vi "Smart_Irrigation_Labview.vi"() -> ()   [LabVIEW 2020]
panel:
  in  "Table Control":string[][](table)
  out "Moisture Sensor":dbl(graph)
  out "Flow Out":bool
  out "Moisture-Level":dbl(knob) scale=0.0..100.0
  out "Water-level Sensor":dbl(graph)
  in  "VISA Resource Port":refnum<visa-resource-name>
  out "PUMP ON":bool
  out "PUMP  OFF":bool
  out "Tank (Liters/sec)":dbl(slide) scale=0.0..100.0
  # "RAGING BULLS"
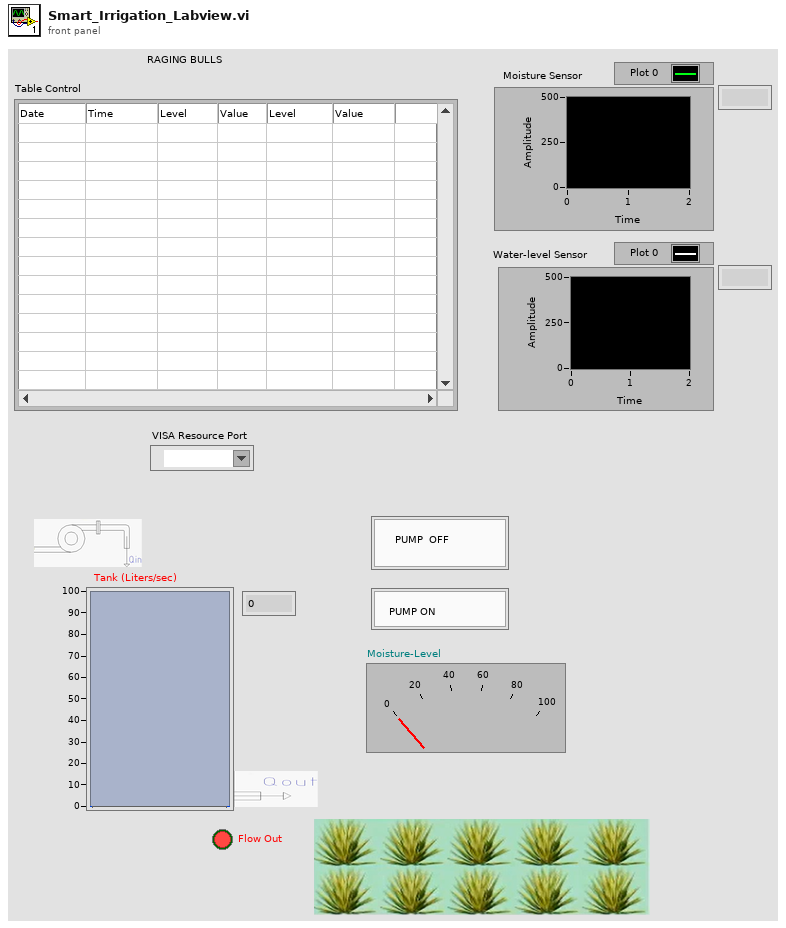
[diagram p1: front panel]
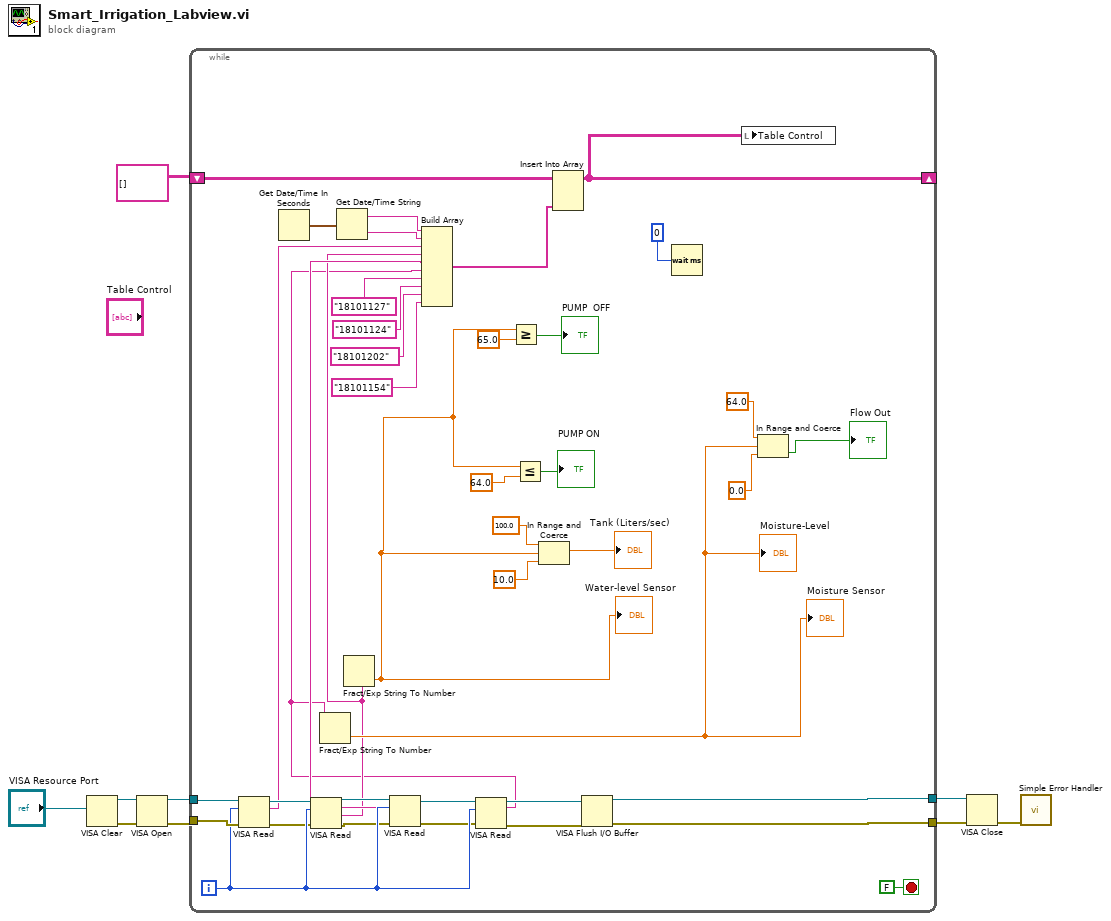
[diagram p0: block diagram]
diagram:
  n1 = VISA Clear(VISA resource name="VISA Resource Port") -> (VISA resource name out=w8:refnum<visa-resource-name>, error out=w9:errorcluster)  [unwired: 1 in]
  n2 = VISA Open(error in (no error)=w9, VISA resource name=w8) -> (VISA resource name=w7:refnum<visa-resource-name>, error out=w6:errorcluster)  [unwired: 3 in]
  n3 = while {
    tunnel: w7 -> [w25]
    tunnel: w6 -> [w24]
    tunnel: [w43] -> w5
    tunnel: [w42] -> w4
    shift-right: [w35] -> _
    shift-left: string[][] [] -> [w36]
    i -> [w23]
    stop <- FALSE stop-if-true
    n4 = VISA Read(VISA resource name=w25, byte count=w23, error in (no error)=w24) -> (VISA resource name out=w26:refnum<visa-resource-name>, read buffer=w17:string, error out=w18:errorcluster)  [unwired: 1 out]
    n5 = Get Date/Time In Seconds() -> (seconds since 1Jan1904=w34:timestamp)
    n6 = VISA Read(VISA resource name=w26, byte count=w23, error in (no error)=w18) -> (VISA resource name out=w22:refnum<visa-resource-name>, read buffer=w15:string, error out=w21:errorcluster)  [unwired: 1 out]
    n7 = Get Date/Time String(seconds (now)=w34) -> (date string=w33:string, time string=w32:string)  [unwired: 2 in]
    n8 = Fract/Exp String To Number(string=w15) -> (number=w30:dbl)  [unwired: 3 in, 1 out]
    "Water-level Sensor" <- w30
    n9 = VISA Read(VISA resource name=w22, byte count=w23, error in (no error)=w21) -> (VISA resource name out=w20:refnum<visa-resource-name>, read buffer=w16:string, error out=w19:errorcluster)  [unwired: 1 out]
    n10 = VISA Read(VISA resource name=w20, byte count=w23, error in (no error)=w19) -> (VISA resource name out=w45:refnum<visa-resource-name>, read buffer=w14:string, error out=w44:errorcluster)  [unwired: 1 out]
    n11 = Fract/Exp String To Number(string=w14) -> (number=w38:dbl)  [unwired: 3 in, 1 out]
    "Moisture-Level" <- w38
    "Moisture Sensor" <- w38
    n12 = Build Array(w33, w32, w17, w15, w16, w14, "18101127" ("element"), "18101124" ("element"), "18101202" ("element"), "18101154" ("element")) -> (w31:string[])
    n13 = Greater Or Equal?(x=w30, y=65.0) -> (x >= y?=→"PUMP  OFF":bool)
    n14 = Less Or Equal?(x=w30, y=64.0) -> (x <= y?=→"PUMP ON":bool)
    n15 = In Range and Coerce(upper limit=100.0, x=w30, lower limit=10.0) -> (coerced(x)=→"Tank (Liters/sec)":dbl)  [unwired: 1 out]
    n16 = Insert Into Array(array=w36, new element=w31) -> (w35:string[][])  [unwired: 2 in]
    n17 = VISA Flush I/O Buffer(VISA resource name=w45, error in (no error)=w44) -> (VISA resource name out=w43:refnum<visa-resource-name>, error out=w42:errorcluster)  [unwired: 1 in]
    n18 = Wait (ms)(milliseconds to wait=u32 0) -> ()  [unwired: 1 out]
    n19 = local write "Table Control"(w35) -> ()
    n20 = In Range and Coerce(upper limit=64.0, x=w38, lower limit=0.0) -> (In Range?=→"Flow Out":bool)  [unwired: 1 out]
  }
  n21 = VISA Close(VISA resource name=w5, error in (no error)=w4) -> (error out=w2:errorcluster)
  n22 = call <vilib>:"Simple Error Handler.vi"("error in (no error)"=w2) -> ()  [unwired: 4 in, 5 out]
